vi "rs3 release frame.vi"(8 "error in (no error)":errorcluster, 10 "Frame":u32, 11 "Device":u32) -> (0 "error out":errorcluster, 1 "error":u64, 3 "Device out":u32)   [LabVIEW 2023]
doc: "You MUST release the FRAME handle soon after you are done with it. It does not have to be immediately, but within about 15 frames."
panel:
  # "RS3 Release Frame"
  # "(C) Intel Corp. 2017,  AGJ"
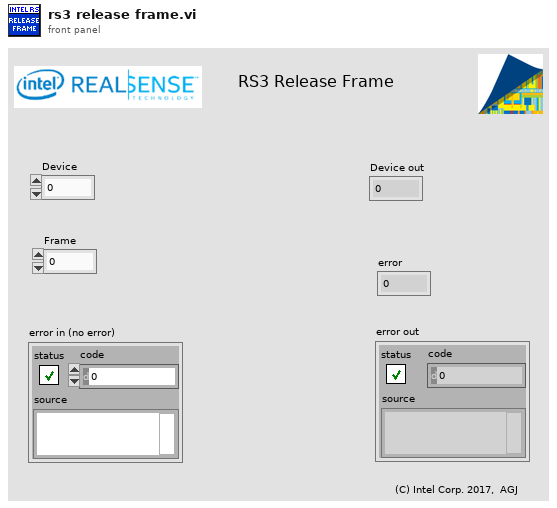
[diagram p1: front panel]
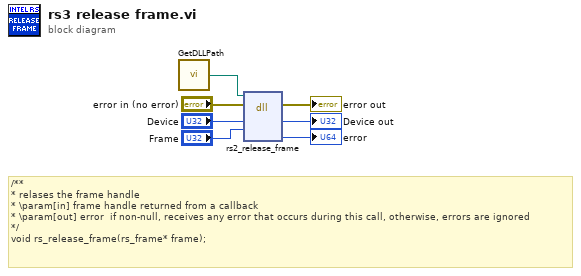
[diagram p0: block diagram]
diagram:
  # "/**\n* relases the frame handle\n* \\param[in] frame handle returned from a callback\n* \\param[out] error  if non-null, receives any error that occurs during this call, otherwise, errors are ignored\n*/\nvoid rs_release_frame(rs_frame* frame);"
  n1 = call "GetDLLPath.vi"() -> ("DLL Path"=w1:path)
  n2 = dll-call lib="C:/STEAMSyndicate/RealSenseWrappers/VI Wrappers (add ons) Public/RealSense/realsense2.dll" fn="rs2_release_frame"(path in=w1, error in="error in (no error)", "device"="Device", "frame"="Frame") -> (error out=→"error out":errorcluster, "device"=→"Device out":u64, "error"=→"error":u64)  [unwired: 4 in, 1 out]
